vi "optionsAcq_channel_gainOffsetAuto.vi"(8 "error in (no error)":errorcluster, 9 "readWrite":enum16{"read", "write"}(ring), 10 "auto":bool, 11 "OSAchannel in":refnum<class "OSAchannel.lvclass">) -> (0 "error out":errorcluster, 2 "auto read":bool, 3 "OSAchannel out":refnum<class "OSAchannel.lvclass">, 4 "FTSLib_status":i32)   [LabVIEW 2010, in "OSAchannel.lvclass"]
uses:
  OSAchannel.lvclass
  OSAchannel.lvclass/OSAchannel.ctl
  _dll/LVLib/FTSLib.lvlib
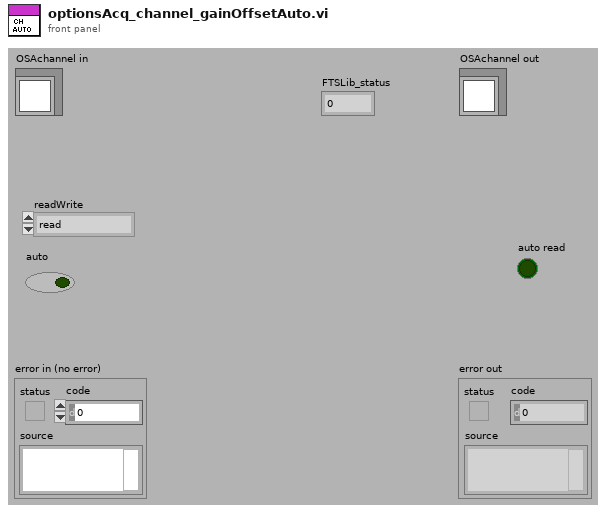
[diagram p1: front panel]
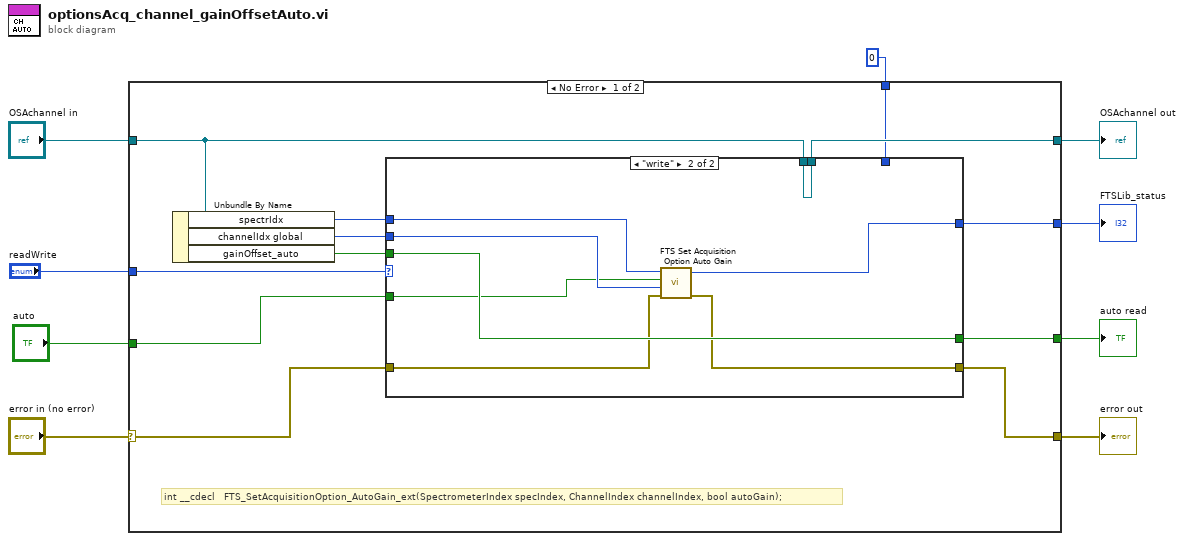
[diagram p0: block diagram]
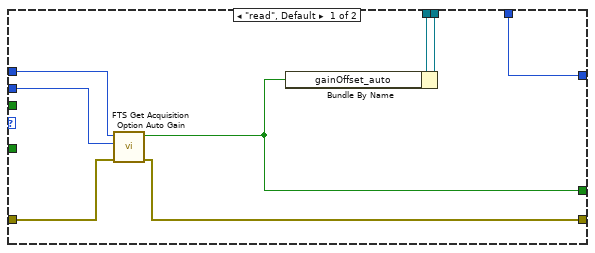
[diagram p2: hidden frame]
diagram:
  n1 = case shown="No Error" "error in (no error)" {
    selector: "error in (no error)" -> [w15 w41]
    tunnel: [w14 w41] -> w8
    tunnel: [w12 w40] -> w6
    tunnel: "OSAchannel in" -> [w13 w40]
    tunnel: "readWrite" -> [w19 _]
    tunnel: "auto" -> [w18 w39]
    tunnel: [w17 w39] -> w3
    tunnel: [w16 w38] -> w2
    tunnel: 0 ("status") -> [w11 w38]
    frame No Error {
      # "int __cdecl   FTS_SetAcquisitionOption_AutoGain_ext(SpectrometerIndex specIndex, ChannelIndex channelIndex, bool autoGain);"
      n2 = Unbundle By Name(w13) -> ("spectrIdx"=w21:u16, "channelIdx global"=w20:u16, "gainOffset_auto"=w10:bool)
      n3 = case shown="\"write\"" w19 {
        tunnel: w21 -> [w24 w33]
        tunnel: w20 -> [w23 w32]
        tunnel: w18 -> [_ w31]
        tunnel: [w22 w36] -> w17
        tunnel: [w27 w30] -> w16
        tunnel: w15 -> [w26 w35]
        tunnel: [w25 w34] -> w14
        tunnel: w13 -> [w29 w37]
        tunnel: [w28 w37] -> w12
        tunnel: w11 -> [w27 _]
        tunnel: w10 -> [_ w36]
        frame "read", Default {
          n4 = call "FTS Get Acquisition Option Auto Gain.vi"("error in (no error)"=w26, "channel"=w23, "specIndex"=w24) -> ("error out"=w25:errorcluster, "function return"=w22:bool)  [unwired: 7 in]
          n5 = Bundle By Name(cluster=w29, "gainOffset_auto"=w22) -> (w28:refnum<class "OSAchannel.lvclass">)
        }
        frame "write" {
          n6 = call "FTS Set Acquisition Option Auto Gain.vi"("error in (no error)"=w35, "channel"=w32, "autoGain"=w31, "specIndex"=w33) -> ("error out"=w34:errorcluster, "function return"=w30:i32)  [unwired: 6 in]
        }
      }
    }
    frame Error {
    }
  }
  "error out" <- w8
  "OSAchannel out" <- w6
  "auto read" <- w3
  "FTSLib_status" <- w2
